vi "Batch Do.vi"(7 "Priority":u16, 8 "error in (no error)":errorcluster, 9 "Message Array in":refnum<class "Message.lvclass">[](array[class]), 10 "Sequencer in":refnum<class "Sequencer.lvclass">, 11 "Batch Msg":refnum<class "Batch Msg.lvclass">) -> (0 "error out":errorcluster, 2 "Sequencer out":refnum<class "Sequencer.lvclass">)   [LabVIEW 2020, in "Sequencer.lvlib" / "Batch Msg.lvclass"]
doc: "Act on the Batch message array.\n\nThe default implementation enqueues the message array in front on the Sequencer Core."
uses:
  Batch Msg.lvclass
  PPL/HDH.Actor Framework.Core.Actor.lvlibp/1abvi3w/vi.lib/ActorFramework/Message/Message.lvclass
  Sequencer/Sequencer.lvclass
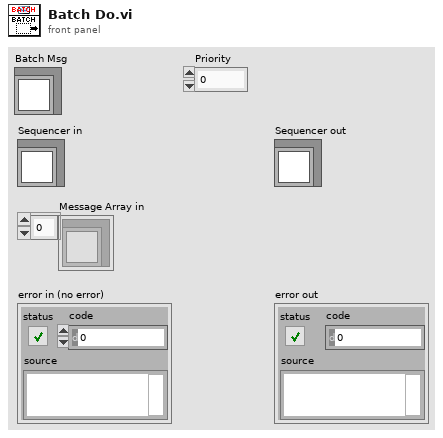
[diagram p1: front panel]
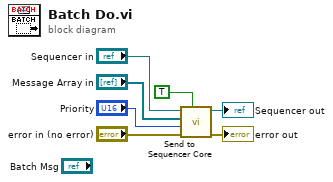
[diagram p0: block diagram]
diagram:
  n1 = call "Send to Sequencer Core.vi"("In Front?(F)"=TRUE, "error in (no error)"="error in (no error)", "Message Priority"="Priority", "Message Array"="Message Array in", "Sequencer in"="Sequencer in") -> ("error out"=→"error out":errorcluster, "Sequencer out"=→"Sequencer out":refnum<class "Sequencer.lvclass">)  [unwired: 5 in]
